vi "Synchronize Control Panel.vi"(8 "error in (no error)":errorcluster, 11 "Neocera LTC-21 in":refnum<class "Neocera LTC-21.lvclass">) -> (0 "error out":errorcluster, 3 "Neocera LTC-21 out":refnum<class "Neocera LTC-21.lvclass">)   [LabVIEW 2015, in "Neocera LTC-21.lvclass"]
uses:
  Neocera LTC-21.lvclass
  Neocera Front Panel Data.ctl
  Neocera Heater Ranges.ctl
  Neocera Set Point Aproach.ctl
  Instrument/Read VISA Resource.vi
  Instrument/Write VISA Resource.vi
  OO Devices/Device/Device.lvclass
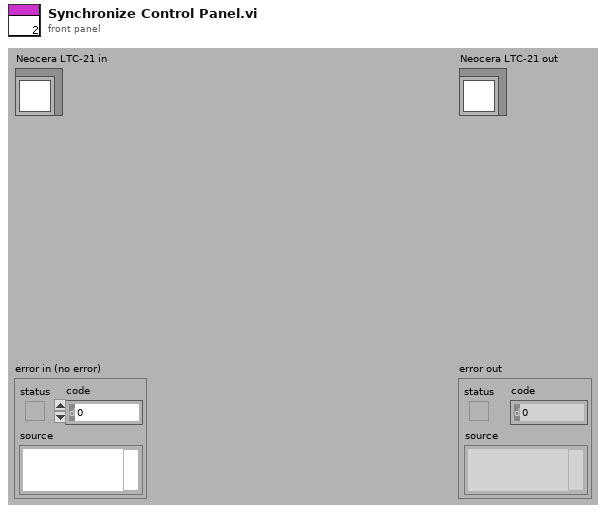
[diagram p1: front panel]
types:
  T1 = typedef "Neocera Front Panel Data.ctl" = cluster{"Channels to measure":dbl[], "Record heater":bool, "Set point":dbl, "Set Heater Range":T2, "Control":bool, "Approach":T3, "Ramp rate, K/min":dbl, "Control Channel":i16, "P":dbl, "I":dbl, "D":dbl, "Suspend heater":bool}
  T2 = typedef "Neocera Heater Ranges.ctl" = enum16{"Off", "0.05W", "0.5W", "5W", "50W"}
  T3 = typedef "Neocera Set Point Aproach.ctl" = enum16{"Instant", "Ramp"}
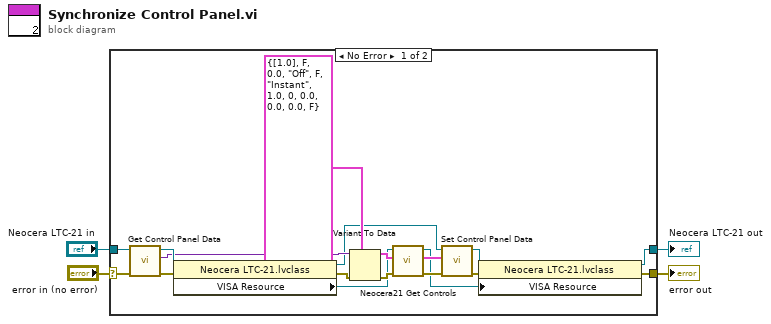
[diagram p0: block diagram]
diagram:
  n1 = case shown="No Error" "error in (no error)" {
    selector: "error in (no error)" -> [w19 w24]
    tunnel: [w11 w24] -> w3
    tunnel: [w7 w23] -> w1
    tunnel: "Neocera LTC-21 in" -> [w22 w23]
    frame No Error {
      n2 = call-dynamic "Get Control Panel Data.vi"("error in (no error)"=w19, "Device in"=w22) -> ("error out"=w13:errorcluster, "Data"=w16:variant, "Device out"=w21:refnum<class "Neocera LTC-21.lvclass">)  [unwired: 7 in]
      n3 = property class="Neocera LTC-21.lvclass"(reference=w21, error in=w13) -> (reference out=w10:refnum<class "Neocera LTC-21.lvclass">, error out=w12:errorcluster, "VISA Resource"=w5:refnum<visa-resource-name>)
      n4 = Variant To Data(error in=w12, type=T1 {"Channels to measure"=[1.0], "Record heater"=FALSE, "Set point"=0.0, "Set Heater Range"=enum."Off", "Control"=FALSE, "Approach"=enum."Instant", "Ramp rate, K/min"=1.0, "Control Channel"=0, "P"=0.0, "I"=0.0, "D"=0.0, "Suspend heater"=FALSE} ("Front Panel Data"), Variant=w16) -> (data=w17:T1, error out=w18:errorcluster)
      n5 = call "Neocera21 Get Controls.vi"("error in (no error)"=w18, "Control Panel Data"=w17, "VISA resource name"=w5) -> ("error out"=w15:errorcluster, "Control Panel Data Out"=w14:T1, "VISA Resource Name Out"=w6:refnum<visa-resource-name>)  [unwired: 6 in]
      n6 = call "Set Control Panel Data.vi"("error in (no error)"=w15, "Data"=w14, "Device in"=w10) -> ("error out"=w8:errorcluster, "Device out"=w9:refnum<class "Neocera LTC-21.lvclass">)  [unwired: 7 in]
      n7 = property class="Neocera LTC-21.lvclass"(reference=w9, error in=w8, "VISA Resource"=w6) -> (reference out=w7:refnum<class "Neocera LTC-21.lvclass">, error out=w11:errorcluster)
    }
    frame Error {
    }
  }
  "error out" <- w3
  "Neocera LTC-21 out" <- w1
